vi "new Door.vi"(8 "error in (no error)":errorcluster) -> (0 "error out":errorcluster, 3 "Door out":refnum<class "Door.lvclass">)   [LabVIEW 2016, in "Door.lvclass"]
uses:
  Door.lvclass
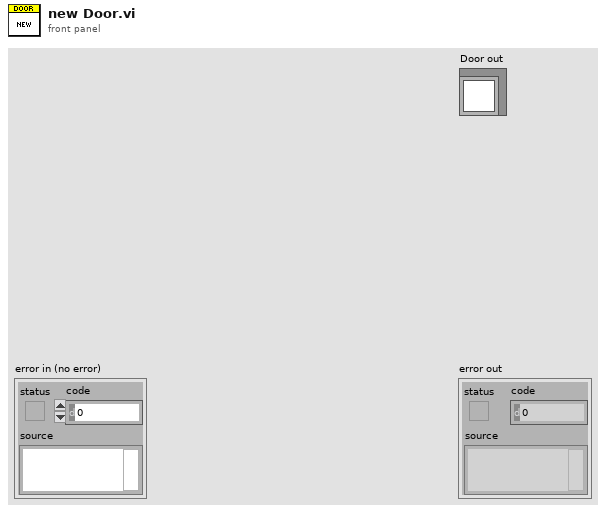
[diagram p1: front panel]
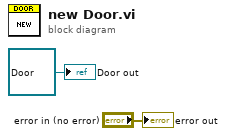
[diagram p0: block diagram]
diagram:
  "error out" <- "error in (no error)"
  "Door out" <- refnum<class "Door.lvclass"> refnum ("Door in")
